vi "Pneumatic Control Initialize.vi"(9 "Forward?":bool, 10 "SolenoidDevRef":T1, 11 "name (unnamed)":string) -> (2 "Sense Loop":T5, 3 "Control Loop":T3)   [LabVIEW 2015]
uses:
  <userlib>/836-Library/Pneumatics/Support Code/Pneumatic Sensor Loop.ctl
  <userlib>/836-Library/Pneumatics/Support Code/Pneumatics Status.ctl
  <vilib>/Rock Robotics/WPI/Solenoid/WPI_SolenoidValue.ctl
  <userlib>/836-Library/Pneumatics/Support Code/Solenoid Control Loop.ctl
  <userlib>/836-Library/Pneumatics/Support Code/Pneumatics Command.ctl
  <userlib>/836-Library/Pneumatics/Support Code/Pneumatics Position.ctl
  <vilib>/Rock Robotics/WPI/Solenoid/WPI_SolenoidDevRef.ctl
  <vilib>/Rock Robotics/WPI/Solenoid/WPI_SolenoidChannel.ctl
  <vilib>/Rock Robotics/WPI/Solenoid/WPI_SolenoidSetEnum.vi
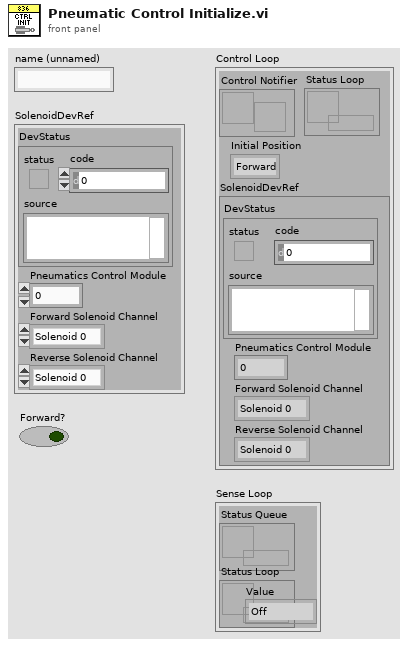
[diagram p1: front panel]
types:
  T1 = typedef "WPI_SolenoidDevRef.ctl" = cluster{"DevStatus":errorcluster, "Pneumatics Control Module":u8, "Forward Solenoid Channel":T2, "Reverse Solenoid Channel":T2}
  T2 = typedef "WPI_SolenoidChannel.ctl" = enum8{"Solenoid 0", "Solenoid 1", "Solenoid 2", "Solenoid 3", "Solenoid 4", "Solenoid 5", "Solenoid 6", "Solenoid 7", "Invalid"}
  T3 = typedef "Solenoid Control Loop.ctl" = cluster{"Control Notifier":refnum<notifier>, "Initial Position":T4, "SolenoidDevRef":T1, "Status Loop":refnum<k33>}
  T4 = typedef "Pneumatics Position.ctl" = enum16{"Forward", "Reverse"}
  T5 = typedef "Pneumatic Sensor Loop.ctl" = cluster{"Status Queue":refnum<queue>, "Status Loop":refnum<k33>, "Relay Value":T6}
  T6 = typedef "WPI_SolenoidValue.ctl" = enum16{"Off", "On", "Forward", "Reverse"}
  T7 = typedef "Pneumatics Command.ctl" = enum16{"Nothing", "Forward", "Reverse", "Toggle"}
  T8 = typedef "Pneumatics Status.ctl" = enum16{"Forward", "Reverse", "Moving"}
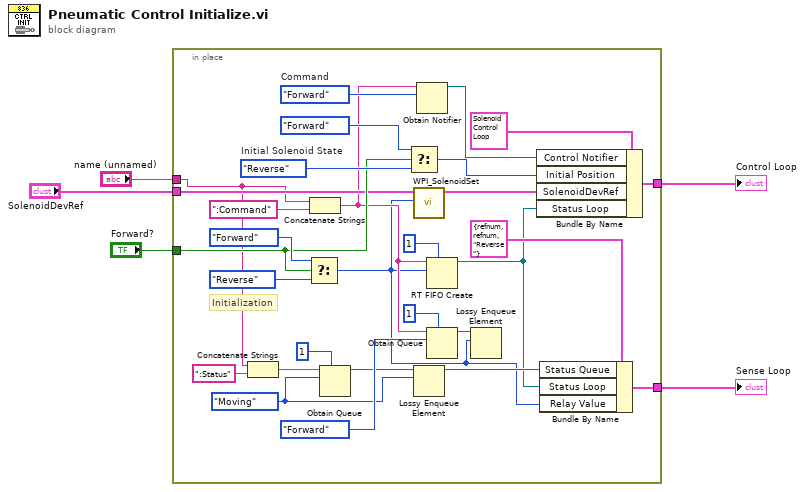
[diagram p0: block diagram]
diagram:
  n1 = in-place {
    in-place-border: "name (unnamed)" -> [w23]
    in-place-border: "Forward?" -> [w30]
    in-place-border: "SolenoidDevRef" -> [w29]
    in-place-border: [w14] -> w4
    in-place-border: [w11] -> w5
    w19 = Pneumatics_Command."Forward"  # Command
    w21 = Pneumatics_Status."Moving" ("Enum")
    w34 = Pneumatics_Position."Reverse"  # Initial Solenoid State
    # "Initialization"
    n2 = Concatenate Strings(w23, ":Status" ("string")) -> (w22:string)
    n3 = Select(t=WPI_SolenoidValue."Forward", s=w30, f=WPI_SolenoidValue."Reverse" ("Value")) -> (s? t:f=w6:T6)
    n4 = Concatenate Strings(w23, ":Command" ("string")) -> (w9:string)
    n5 = Obtain Queue(max queue size (-1, unlimited)=1, name (unnamed)=w22, element data type=w21) -> (queue out=w12:refnum<queue>)  [unwired: 2 in, 2 out]
    n6 = Select(t=Pneumatics_Position."Forward", s=w30, f=w34) -> (s? t:f=w16:T4)
    n7 = call-poly <vilib>:"WPI_SolenoidSet.vi"("Value"=w6, "SolenoidDevRef"=w29) -> ("SolenoidDevRef"=w15:T1)  [unwired: 8 in, 1 out]
    n8 = Lossy Enqueue Element(queue=w12, element=w21) -> (queue out=w10:refnum<queue>)  [unwired: 1 in, 3 out]
    n9 = Obtain Notifier(name (unnamed)=w9, notification data type=w19) -> (notifier out=w17:refnum<notifier>)  [unwired: 2 in, 2 out]
    n10 = RT FIFO Create(0:w9, 1:w6, 4:u32 1 ("size (10)")) -> (8:w8:refnum<k33>)  [unwired: 5 in, 2 out]
    n11 = Obtain Queue(max queue size (-1, unlimited)=1, name (unnamed)=w9, element data type=WPI_SolenoidValue."Forward" ("Value")) -> (queue out=w27:refnum<queue>)  [unwired: 2 in, 2 out]
    n12 = Lossy Enqueue Element(queue=w27, element=w6) -> ()  [unwired: 1 in, 4 out]
    n13 = Bundle By Name(cluster=T3 {"Control Notifier"=refnum, "Initial Position"=enum."Forward", "SolenoidDevRef"={"DevStatus"={"status"=FALSE, "code"=0, "source"=""}, "Pneumatics Control Module"=0, "Forward Solenoid Channel"=enum."Invalid", "Reverse Solenoid Channel"=enum."Invalid"}, "Status Loop"=refnum}, "Control Notifier"=w17, "Initial Position"=w16, "SolenoidDevRef"=w15, "Status Loop"=w8) -> (w14:T3)
    n14 = Bundle By Name(cluster=T5 {"Status Queue"=refnum, "Status Loop"=refnum, "Relay Value"=enum."Reverse"}, "Status Queue"=w10, "Status Loop"=w8, "Relay Value"=w6) -> (w11:T5)
  }
  "Sense Loop" <- w5
  "Control Loop" <- w4
